vi "API - Continuous Capture - Capture Continuously.vi"(7 "Maximum Caputre Rate (Full Buffers/Second)":i32=1000, 8 "error in":errorcluster, 9 "Data Size":T1, 10 "Buffer Block Size (Samples/Channel)":i32=256, 11 "Configuration file path":path) -> (0 "error out":errorcluster)   [LabVIEW 2017, in "DTACQ - Network Enabled Device Driver.lvlib"]
doc: "Continuously captures data from the device and publishes that data to shared variables.\nThe while loop will continue infinitely, unless;\n-An error is encountered\n-Another VI executes the close command. \n(Causes an error in the fetch data command, which in turn causes the loop to terminate.)"
uses:
  DTACQ - Network Enabled Device Driver.lvlib
  Communications/Typedefs/Data Size--Enum.ctl
  Close Continuous Mode.vi
  Read Continuous Data and Write to Shared Variable.vi
  Initialise Continuous Capture Mode.vi
  Communications/Communications Library.lvlib
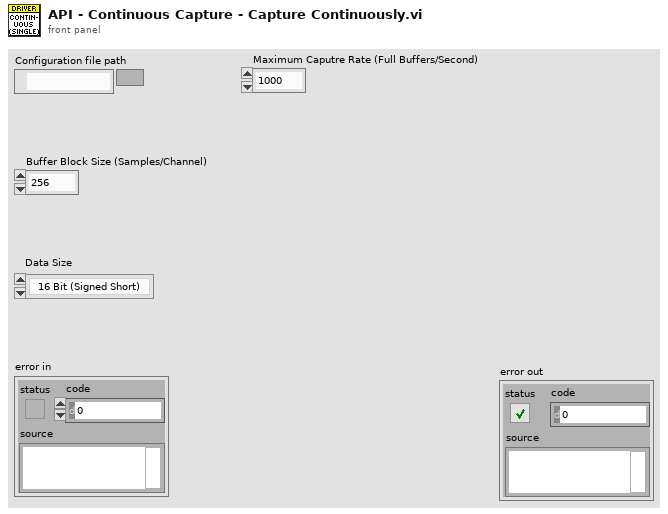
[diagram p1: front panel]
types:
  T1 = typedef "Communications Library.lvlib/Data Size--Enum.ctl" = enum16{"16 Bit (Signed Short)", "32 Bit (Signed Long)"}
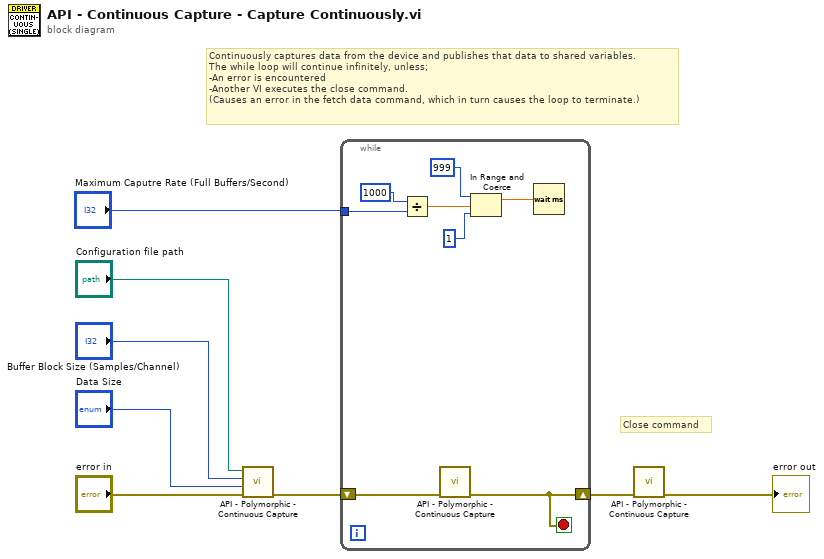
[diagram p0: block diagram]
diagram:
  # "Close command"
  # "Continuously captures data from the device and publishes that data to shared variables.\nThe while loop will continue infinitely, unless;\n-An error is encountered\n-Another VI executes the close command. \n(Causes an error in the fetch data command, which in turn causes the loop to terminate.)"
  n1 = call-poly "API - Polymorphic - Continuous Capture.vi"("error in"="error in", "Data Size"="Data Size", "Buffer Block Size (Samples/Channel)"="Buffer Block Size (Samples/Channel)", "configuration file path"="Configuration file path") -> ("error out"=w4:errorcluster)  [unwired: 7 in]
  n2 = while {
    shift-right: [w9] -> w3
    shift-left: w4 -> [w16]
    tunnel: "Maximum Caputre Rate (Full Buffers/Second)" -> [w11]
    stop <- w9 stop-if-true
    n3 = Divide(x=1000 ("y"), y=w11) -> (x/y=w10:dbl)
    n4 = call-poly "API - Polymorphic - Continuous Capture.vi"("error in"=w16) -> ("error out"=w9:errorcluster)  [unwired: 10 in]
    n5 = In Range and Coerce(upper limit=999, x=w10, lower limit=1 ("upper limit")) -> (coerced(x)=w15:dbl)  [unwired: 1 out]
    n6 = Wait (ms)(milliseconds to wait=w15) -> ()  [unwired: 1 out]
  }
  n7 = call-poly "API - Polymorphic - Continuous Capture.vi"("error in"=w3) -> ("error out"=→"error out":errorcluster)  [unwired: 10 in]
